vi "JoystickHelp.vi"() -> ()   [LabVIEW 2014]
panel:
  out "String":string="The Joystick Direction plot shows the joystick deflection in X and Y direction. A small cross shows the current deflection and a red trace shows the history for the last few seconds.\n\nThe Vertical Thruster Allocation shows the gain sent to the ROV to adjust the heave position. \n\nThe Yaw Thruster Allocation shows the gain sent to the ROV to adjust the yaw position\n\nThe joystick selector determine which joystick connected to the system to be used. It can be changed during run-time.\n\nThe POV Direction shows the direction of the rubber hat direction switch on the top of the joystick.\n\nThe joystick mode have three main modes:\n- Manual Thrust Allocation\n- Position Reference\n- Velocity Reference\n\nFor the two latter modes the frame can be selected between:\n- Body\n- NED\n\n"
  out "2D Picture":picture
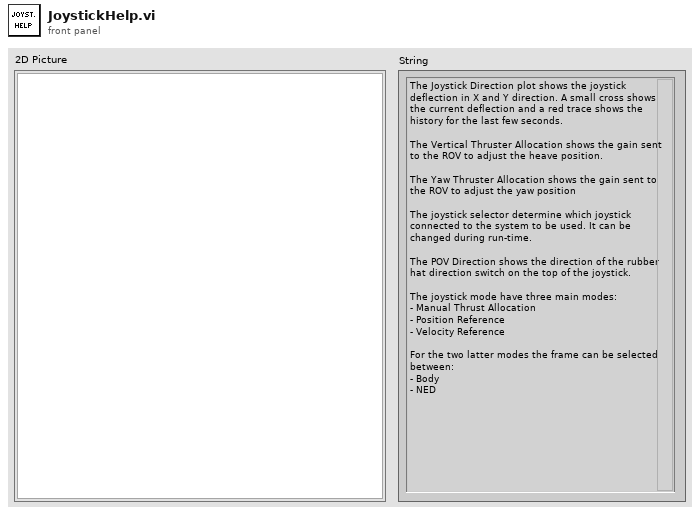
[diagram p1: front panel]
types:
  T1 = typedef "imagedata.ctl" = cluster{"image type":i32, "image depth":i32, "image":u8[], "mask":u8[], "colors":u32[], "Rectangle":cluster{"left":i16, "top":i16, "right":i16, "bottom":i16}}
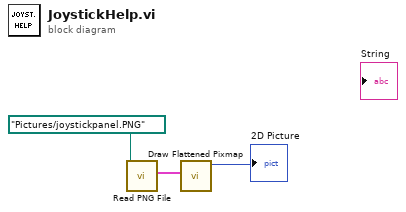
[diagram p0: block diagram]
diagram:
  n1 = call <vilib>:"Read PNG File.vi"("path to PNG file"=path "Pictures/joystickpanel.PNG") -> ("image data"=w2:T1)  [unwired: 8 in, 2 out]
  n2 = call <vilib>:"Draw Flattened Pixmap.vi"("image data"=w2) -> ("new picture"=→"2D Picture":picture)  [unwired: 8 in]
